vi "DK240 WaveInfo.vi"(5 "error in":errorcluster, 6 "Port":refnum<visa-resource-name>="SPECTRO") -> (0 "error out":errorcluster, 2 "Status":u8, 3 "Wavelenght":dbl caption="Longueur \nd'onde (nm)" min=0.0 max=167770.0 step=1.0 format="%#.2f")   [LabVIEW 2019]
doc: "Ce VI retourne la longueur d'ondes actuel.\n\nThis VI returns the current wavelength."
uses:
  <vilib>/Utility/error.llb/DialogType.ctl
panel:
  out "Cancel":u8
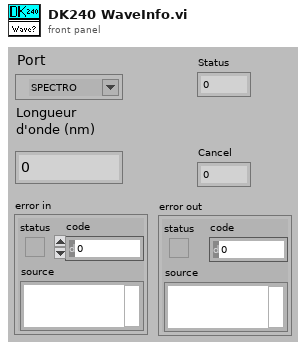
[diagram p1: front panel]
types:
  T1 = typedef "DialogType.ctl" = u16
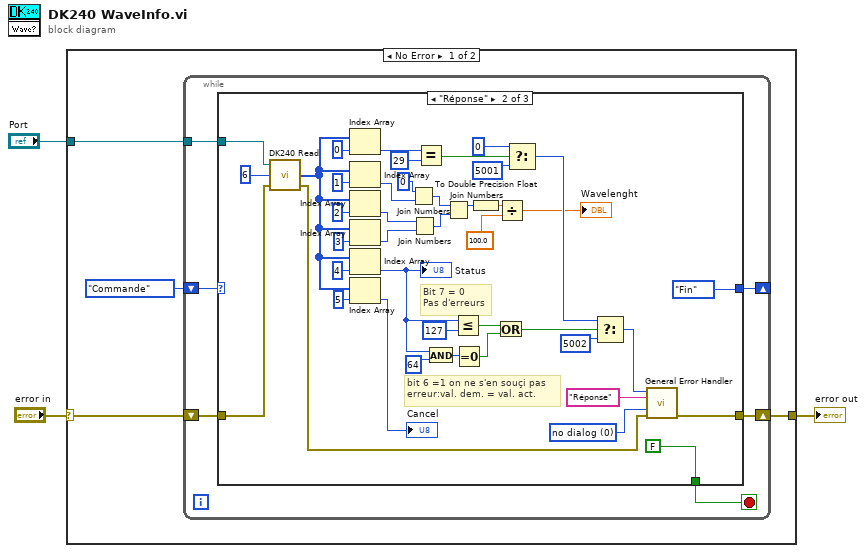
[diagram p0: block diagram]
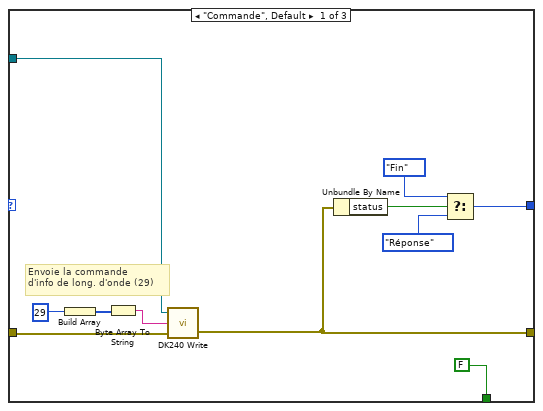
[diagram p2: hidden frame]
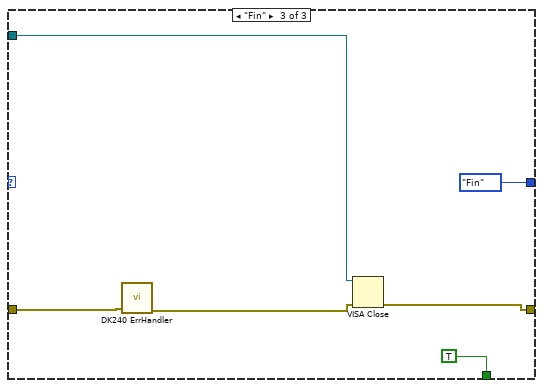
[diagram p3: hidden frame]
diagram:
  n1 = case shown="No Error" "error in" {
    selector: "error in" -> [w4 w73]
    tunnel: "Port" -> [w7 _]
    tunnel: [w6 w73] -> w1
    frame No Error {
      n2 = while {
        tunnel: w7 -> [w12]
        shift-right: [w10] -> w6
        shift-left: w4 -> [w11]
        shift-right: [w8] -> _
        shift-left: enum16{"Commande", "Réponse", "Fin"}."Commande" -> [w9]
        stop <- w13 stop-if-true
        n3 = case shown="\"Réponse\"" w9 {
          tunnel: [FALSE FALSE TRUE] -> w13
          tunnel: w12 -> [w20 w60 w69]
          tunnel: w11 -> [w19 w59 w68]
          tunnel: [w16 w47 w70] -> w10
          tunnel: [w14 enum16{"Commande", "Réponse", "Fin"}."Fin" enum16{"Commande", "Réponse", "Fin"}."Fin"] -> w8
          frame "Commande", Default {
            # "Envoie la commande\nd'info de long. d'onde (29)"
            n4 = Build Array(u8 29) -> (w24:u8[])
            n5 = Byte Array To String(unsigned byte array=w24) -> (string=w21:string)
            n6 = call <userlib>:"DK240 Write.vi"("error in"=w19, "String to write"=w21, "Port"=w20) -> ("error out"=w16:errorcluster)  [unwired: 1 in]
            n7 = Unbundle By Name(w16) -> ("status"=w15:bool)
            n8 = Select(t=enum16{"Commande", "Réponse", "Fin"}."Fin", s=w15, f=enum16{"Commande", "Réponse", "Fin"}."Réponse") -> (s? t:f=w14:enum16{"Commande", "Réponse", "Fin"})
          }
          frame "Réponse" {
            w53 = T1 0 items=["no dialog", "OK message", "continue or stop message", "OK message + warnings", "continue/stop + warnings"] ("type of dialog (OK msg:1)")
            # "bit 6 =1 on ne s'en souçi pas \nerreur:val. dem. = val. act."
            # "Bit 7 = 0\nPas d'erreurs"
            n9 = call <userlib>:"DK240 Read.vi"("error in"=w59, "Byte count"=u32 6, "Port"=w60) -> ("error out"=w48:errorcluster, "Received Bytes"=w44:u8[])  [unwired: 1 in]
            n10 = Index Array(array=w44, index=0) -> (element=w40:u8)
            n11 = Index Array(array=w44, index=1) -> (element=w36:u8)
            n12 = Index Array(array=w44, index=2) -> (element=w33:u8)
            n13 = Index Array(array=w44, index=3) -> (element=w32:u8)
            n14 = Index Array(array=w44, index=4) -> (element=w34:u8)
            "Status" <- w34
            n15 = Index Array(array=w44, index=5) -> (element=→"Cancel":u8)
            n16 = Join Numbers(hi=u8 0, lo=w36) -> ((hi.lo)=w28:u16)
            n17 = Join Numbers(hi=w33, lo=w32) -> ((hi.lo)=w27:u16)
            n18 = Equal?(x=w40, y=u8 29) -> (x = y?=w38:bool)
            n19 = And(x=w34, y=u8 64) -> (x .and. y?=w55:u8)
            n20 = Join Numbers(hi=w28, lo=w27) -> ((hi.lo)=w30:u32)
            n21 = Less Or Equal?(x=w34, y=u8 127) -> (x <= y?=w56:bool)
            n22 = Equal To 0?(x=w55) -> (x = 0?=w57:bool)
            n23 = To Double Precision Float(number=w30) -> (double precision float=w26:dbl)
            n24 = Or(x=w56, y=w57) -> (x .or. y?=w58:bool)
            n25 = Divide(x=w26, y=100.0) -> (x/y=→"Wavelenght":dbl)
            n26 = Select(t=0, s=w38, f=5001 ("t")) -> (s? t:f=w37:i32)
            n27 = Select(t=w37, s=w58, f=5002 ("t")) -> (s? t:f=w50:i32)
            n28 = call <vilib>:"General Error Handler.vi"("[error code] (0)"=w50, "[error source] (\" \")"="Réponse" ("[error source] (\" \")"), "type of dialog (OK msg:1)"=w53, "error in (no error)"=w48) -> ("error out"=w47:errorcluster)  [unwired: 7 in, 4 out]
          }
          frame "Fin" {
            n29 = call <userlib>:"DK240 ErrHandler.vi"("error in"=w68) -> ("error out"=w67:errorcluster)  [unwired: 7 in]
            n30 = VISA Close(VISA resource name=w69, error in (no error)=w67) -> (error out=w70:errorcluster)
          }
        }
      }
    }
    frame Error {
    }
  }
  "error out" <- w1
